vi "Path to URL.vi"(1 "path":path) -> (0 "url":string)   [LabVIEW 2020]
panel:
  # "Please do not change label names on this VI -- they are used by VI Server in runtime applications."
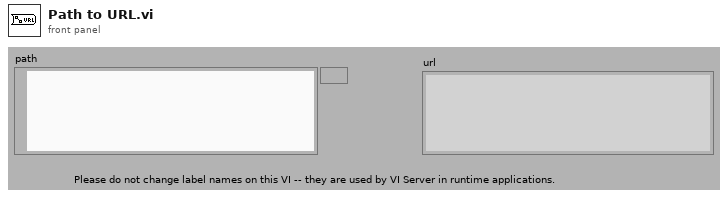
[diagram p1: front panel]
types:
  T1 = enum32{"invalid OS target", "Mac OS", "Windows 3.1", "Windows 95/NT", "Solaris 1", "Solaris 2", "HP-UX", "PowerMAX", "Linux", "Irix", "Rhapsody", "BeOS", "AIX", "OSF1", "VxWorks", "PharLap", "Carbon", "RTX", "Windows x64", "Linux x64", "Mac OS X x64"}
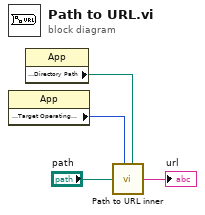
[diagram p0: block diagram]
diagram:
  n1 = property class="App"() -> ("Application:Target Operating System"=w3:T1)  [unwired: 2 in, 2 out]
  n2 = property class="App"() -> ("Application:Directory Path"=w1:path)  [unwired: 2 in, 2 out]
  n3 = call "Path to URL inner.vi"("path"="path", "App.TargetOS"=w3, "Application:Directory Path"=w1) -> ("url"=→"url":string)
